vi "Connect CAN Adapter.vi"(8 "error in (no error)":errorcluster, 10 "ICommunicate Class Name":string, 11 "CANopen Master in":refnum<class "CANopen Master.lvclass">) -> (0 "error out":errorcluster, 3 "CANopen Master out":refnum<class "CANopen Master.lvclass">)   [LabVIEW 2024, in "CANopen Master.lvlib" / "CANopen Master.lvclass"]
uses:
  CANopen Master/CANopen Master.lvclass
  HAL/Source/Interfaces/ICommunicate/ICommunicate.lvclass
  CANopen Master/CANopen Master.lvclass/CANopen Master.ctl
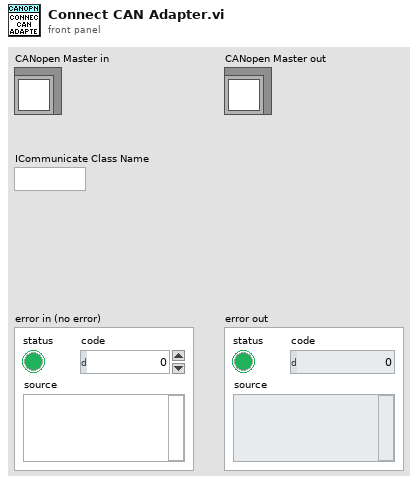
[diagram p1: front panel]
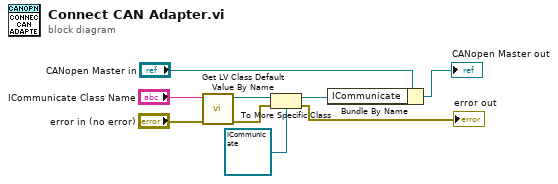
[diagram p0: block diagram]
diagram:
  n1 = call <vilib>:"Get LV Class Default Value By Name.vi"("error in (no error)"="error in (no error)", "class name"="ICommunicate Class Name") -> ("error out"=w8:errorcluster, "object"=w9:refnum<class>)  [unwired: 8 in]
  n2 = To More Specific Class(target class=refnum<class "ICommunicate.lvclass"> refnum ("ICommunicate.lvclass"), reference=w9, error in=w8) -> (specific class reference=w2:refnum<class "ICommunicate.lvclass">, error out=→"error out":errorcluster)
  n3 = Bundle By Name(cluster="CANopen Master in", "ICommunicate"=w2) -> (→"CANopen Master out":refnum<class "CANopen Master.lvclass">)
